vi "read station dio map.vi"(7 "error in":errorcluster, 9 "station idx":i32, 10 "configuration file path in":path) -> (0 "error out":errorcluster, 1 "D in map":T2, 2 "DO Task":refnum<k21>, 3 "configuration file path out":path)   [LabVIEW 2018]
uses:
  02.Type Def's/station DI map.ctl
  05.UserVI's/type defs/EOL Global Digital Input Control.ctl
  05.UserVI's/type defs/EOL Global Digital Output Control.ctl
  05.UserVI's/file io/ini/type defs/ini entry.ctl
  05.UserVI's/file io/ini/type defs/ini entry types.ctl
  05.UserVI's/file io/ini/type defs/ini entry value.ctl
  <vilib>/DAQmx/create/channels.llb/DAQmx Create Channel (DO-Digital Output).vi
panel:
  out "DO":T1
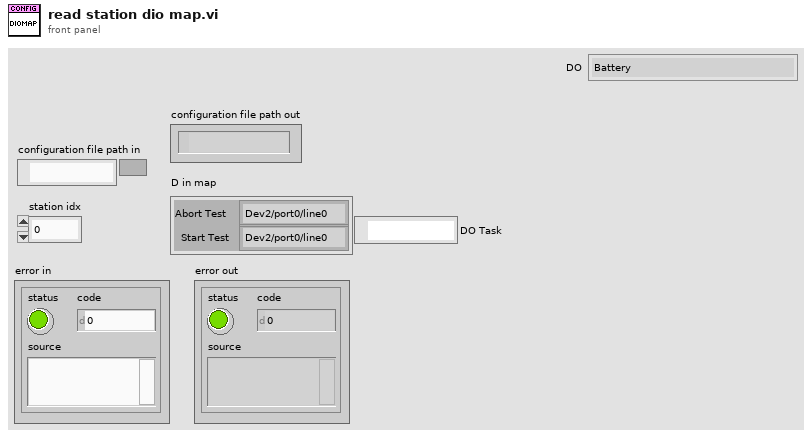
[diagram p1: front panel]
types:
  T1 = typedef "EOL Global Digital Output Control.ctl" = enum16{"Battery", "IGN High", "IGN Low", "LIN", "CAN", "Switch 1", "Switch 2", "Switch 3", "Switch 4", "Switch 5", "Switch 6", "Glass Analog Switch 1", "Glass Analog Switch 2", "Glass Analog Switch 3", "Glass Analog Switch 4", "Sunshade Analog Switch 1", "Sunshade Analog Switch 2", "Sunshade Analog Switch 3", "Sunshade Analog Switch 4", "Glass Motor Relay 1", "Glass Motor Relay 2", "Sunshade Motor Relay 1", "Sunshade Motor Relay 2"}
  T2 = typedef "station DI map.ctl" = cluster{"Abort Test":T3, "Start Test":T3}
  T3 = typedef "EOL Global Digital Input Control.ctl" = enum16{"Dev2/port0/line0", "Dev2/port0/line1", "Dev2/port0/line2", "Dev2/port0/line3", "Dev2/port0/line4", "Dev2/port0/line5", "Dev2/port0/line6", "Dev2/port0/line7", "Dev2/port1/line0", "Dev2/port1/line1", "Dev2/port1/line2", "Dev2/port1/line3", "Dev2/port1/line4", "Dev2/port1/line5", "Dev2/port1/line6", "Dev2/port1/line7", "Dev2/port2/line0", "Dev2/port2/line1", "Dev2/port2/line2", "Dev2/port2/line3", "Dev2/port2/line4", "Dev2/port2/line5", "Dev2/port2/line6", "Dev2/port2/line7", "Prerun Start Test", "Prerun Abort Test", "Audit Start Test", "Audit Abort Test", "Dev2/port3/line4", "Dev2/port3/line5", "Breakin Start Test", "Breakin Abort Test", "Not Implemented"}
  T4 = enum16{"Init", "Write", "Write All", "Clear All", "Stop", "Read"}
  T5 = typedef "ini entry types.ctl" = enum16{"Boolean", "Double", "I32", "Path", "String", "U32"}
  T6 = typedef "ini entry.ctl" = cluster{"section":string, "key":string, "type":T5, "default value":T7}
  T7 = typedef "ini entry value.ctl" = cluster{"Boolean":bool, "Dbl":dbl, "I32":i32, "Path":path, "String":string, "U32":u32}
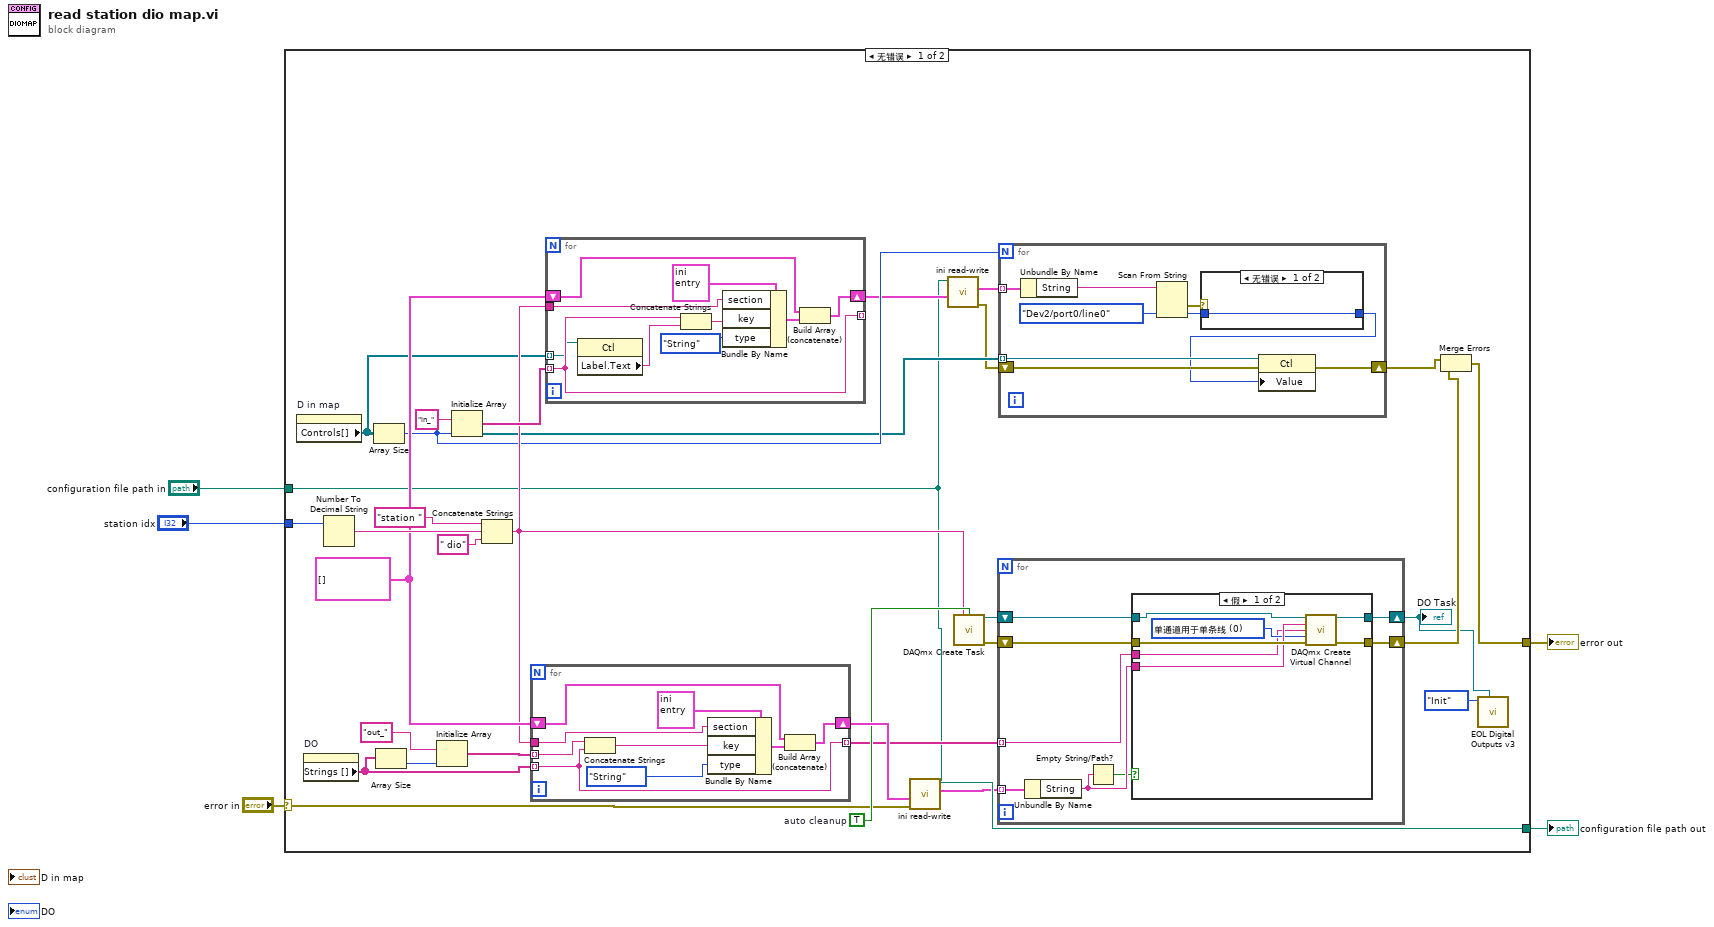
[diagram p0: block diagram]
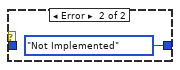
[diagram p2: hidden frame]
diagram:
  n1 = case shown="无错误" "error in" {
    selector: "error in" -> [w12 w85]
    tunnel: "configuration file path in" -> [w13 w84]
    tunnel: [w36 w84] -> w4
    tunnel: [w9 w85] -> w3
    tunnel: "station idx" -> [w34 _]
    frame No Error {
      w25 = TRUE  # auto cleanup
      w20 = T6[] []
      n2 = property on="D in map" class="Clust (严格)"() -> ("Controls[]"=w16:refnum<vi>[])  [unwired: 2 in, 2 out]
      n3 = property on="DO" class="Enum (严格)"() -> ("Strings []"=w21:string[])  [unwired: 2 in, 2 out]
      n4 = Number To Decimal String(number=w34) -> (decimal integer string=w33:string)  [unwired: 1 in]
      n5 = Array Size(array=w16) -> (size(s)=w17:i32)
      n6 = Array Size(array=w21) -> (size(s)=w28:i32)
      n7 = Initialize Array("out_", w28) -> (w26:string[])
      n8 = Initialize Array("in_", w17) -> (w19:string[])
      n9 = Concatenate Strings("station ", w33, " dio") -> (w18:string)
      n10 = for {
        tunnel: w18 -> [w79]
        shift-right: [w82] -> w32
        shift-left: w20 -> [w81]
        tunnel: w26 -> [w76] mode=indexing
        tunnel: [w75] -> w22 mode=indexing
        tunnel: w21 -> [w75] mode=indexing
        n11 = Concatenate Strings(w76, w75) -> (w77:string)
        n12 = Bundle By Name(cluster=T6 {"section"="", "key"="", "type"=enum."Boolean", "default value"={"Boolean"=FALSE, "Dbl"=0.0, "I32"=0, "Path"=path "", "String"="", "U32"=0}}, "section"=w79, "key"=w77, "type"=ini_entry_types."String") -> (w83:T6)
        n13 = Build Array (concatenate)(w81, w83) -> (w82:T6[])
      }
      n14 = for {
        tunnel: w18 -> [w53]
        shift-right: [w56] -> w14
        shift-left: w20 -> [w55]
        tunnel: [w50] -> _ mode=indexing
        tunnel: w19 -> [w50] mode=indexing
        tunnel: w16 -> [w49] mode=indexing
        n15 = property class="Ctl"(reference=w49) -> ("Label.Text"=w48:string)  [unwired: 1 in, 2 out]
        n16 = Concatenate Strings(w50, w48) -> (w51:string)
        n17 = Bundle By Name(cluster=T6 {"section"="", "key"="", "type"=enum."Boolean", "default value"={"Boolean"=FALSE, "Dbl"=0.0, "I32"=0, "Path"=path "", "String"="", "U32"=0}}, "section"=w53, "key"=w51, "type"=ini_entry_types."String") -> (w57:T6)
        n18 = Build Array (concatenate)(w55, w57) -> (w56:T6[])
      }
      n19 = call "ini read-write.vi"("error in (no error)"=w12, "ini entry descriptors"=w32, "configuration file path"=w13) -> ("values out"=w27:T7[], "configuration file path out"=w36:path)  [unwired: 6 in, 1 out]
      n20 = call "ini read-write.vi"("ini entry descriptors"=w14, "configuration file path"=w13) -> ("error out"=w8:errorcluster, "values out"=w15:T7[])  [unwired: 7 in, 1 out]
      n21 = call <vilib>:"DAQmx Create Task.vi"("new task name"=w18, "auto cleanup"=w25) -> ("task out"=w24:refnum<k21>, "error out"=w23:errorcluster)  [unwired: 12 in]
      n22 = for {
        shift-right: [w65] -> w6
        shift-left: w24 -> [w64]
        shift-right: [w62] -> w10
        shift-left: w23 -> [w63]
        tunnel: w27 -> [w61] mode=indexing
        tunnel: w22 -> [w58] mode=indexing
        n23 = Unbundle By Name(w61) -> ("String"=w60:string)
        n24 = Empty String/Path?(string/path=w60) -> (empty?=w59:bool)
        n25 = case shown="假" w59 {
          tunnel: [w72 w74] -> w65
          tunnel: w64 -> [w71 w74]
          tunnel: w63 -> [w70 w73]
          tunnel: [w69 w73] -> w62
          tunnel: w60 -> [w68 _]
          tunnel: w58 -> [w66 _]
          frame False {
            w67 = 0 items=["单通道用于单条线", "单通道用于所有线"] ("line grouping")
            n26 = call-poly <vilib>:"DAQmx Create Virtual Channel.vi"("task in"=w71, "lines"=w68, "name to assign"=w66, "line grouping"=w67, "error in"=w70) -> ("task out"=w72:refnum<k21>, "error out"=w69:errorcluster)  [unwired: 9 in]
          }
          frame True {
          }
        }
      }
      "DO Task" <- w6
      n27 = for {
        N: w17 -> [_]
        tunnel: w15 -> [w40] mode=indexing
        tunnel: w16 -> [w45] mode=indexing
        shift-right: [w44] -> w11
        shift-left: w8 -> [w43]
        n28 = Unbundle By Name(w40) -> ("String"=w42:string)
        n29 = Scan From String(input string=w42, default 1=EOL_Global_Digital_Input_Control."Dev2/port0/line0" ("Abort Test")) -> (error out=w39:errorcluster, output 1=w37:T3)  [unwired: 3 in, 2 out]
        n30 = case shown="无错误" w39 {
          tunnel: [w46 EOL_Global_Digital_Input_Control."Not Implemented" ("Abort Test")] -> w38
          tunnel: w37 -> [w46 _]
          frame No Error {
          }
          frame Error {
          }
        }
        n31 = property class="Ctl"(reference=w45, error in=w43, "Value"=w38) -> (error out=w44:errorcluster)  [unwired: 1 out]
      }
      n32 = Merge Errors(w11, w10) -> (w9:errorcluster)
      n33 = call "EOL Digital Outputs v3.vi"("task/channels in"=w6, "Mode"=T4."Init") -> ()  [unwired: 8 in, 2 out]
    }
    frame Error {
    }
  }
  "configuration file path out" <- w4
  "error out" <- w3
